vi "Control Cluster(SubVI).vi"(10 "Control cluster In New":T1, 11 "Control cluster In Original":T1) -> (3 "Control cluster Out":T1)   [LabVIEW 2014]
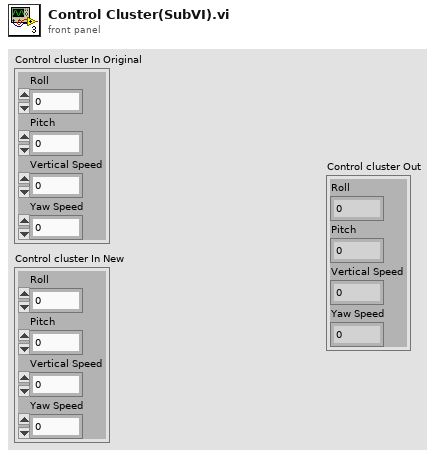
[diagram p1: front panel]
types:
  T1 = cluster{"Roll":dbl, "Pitch":dbl, "Vertical Speed":dbl, "Yaw Speed":dbl}
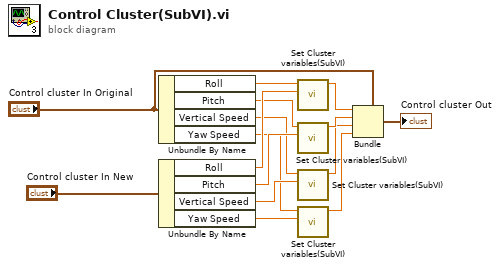
[diagram p0: block diagram]
diagram:
  n1 = Unbundle By Name("Control cluster In Original") -> ("Roll"=w13:dbl, "Pitch"=w10:dbl, "Vertical Speed"=w8:dbl, "Yaw Speed"=w5:dbl)
  n2 = Unbundle By Name("Control cluster In New") -> ("Roll"=w14:dbl, "Pitch"=w9:dbl, "Vertical Speed"=w7:dbl, "Yaw Speed"=w6:dbl)
  n3 = call "Set Cluster variables(SubVI).vi"("Roll 3"=w14, "Roll in"=w13) -> ("Roll out"=w12:dbl)  [unwired: 9 in]
  n4 = call "Set Cluster variables(SubVI).vi"("Roll 3"=w9, "Roll in"=w10) -> ("Roll out"=w4:dbl)  [unwired: 9 in]
  n5 = call "Set Cluster variables(SubVI).vi"("Roll 3"=w7, "Roll in"=w8) -> ("Roll out"=w3:dbl)  [unwired: 9 in]
  n6 = call "Set Cluster variables(SubVI).vi"("Roll 3"=w6, "Roll in"=w5) -> ("Roll out"=w2:dbl)  [unwired: 9 in]
  n7 = Bundle(cluster="Control cluster In Original", "Roll"=w12, "Pitch"=w4, "Vertical Speed"=w3, "Yaw Speed"=w2) -> (→"Control cluster Out":T1)
